vi "Parse JSON Item.vi"(8 "error in (no error)":errorcluster, 9 "Name":string, 10 "Variant in":variant, 11 "JSON In":string) -> (0 "error out":errorcluster, 2 "Variant out":variant)   [LabVIEW 2018]
uses:
  a599c9c2-7984-4765-8e85-315dde484629.vi
  <vilib>/JDP Science/JSONtext/Next JSON Value.vi
  <vilib>/JDP Science/JSONtext/String Subset.vi
  <vilib>/JDP Science/JSONtext/Parsing/Advance past next JSON Value (inlined COPY).vi
  <vilib>/JDP Science/JSONtext/Parsing/Advance past whitespace.vi
  <vilib>/JDP Science/JSONtext/Parsing/Advance past String.vi
  <vilib>/JDP Science/JSONtext/Parsing/Advance past Number.vi
  <vilib>/JDP Science/JSONtext/Parsing/Advance past Line Ending.vi
  <vilib>/JDP Science/JSONtext/Parsing/Parse Full Path or Item Name.vi
  <vilib>/JDP Science/JSONtext/Parsing/Advance past Array.vi
  <vilib>/JDP Science/JSONtext/Parsing/Advance past Object.vi
  <vilib>/JDP Science/JSONtext/support/Error Cluster From Code.vi
  <vilib>/JDP Science/JSONtext/Offset/Find Item Locations by Path.vi
  <vilib>/JDP Science/JSONtext/JSON text to Variant.vi
  <vilib>/JDP Science/JSONtext/LVClass Serializer/JSONtext LVClass Serializer.lvclass
  <vilib>/JDP Science/JSONtext/JSONtext.lvlib
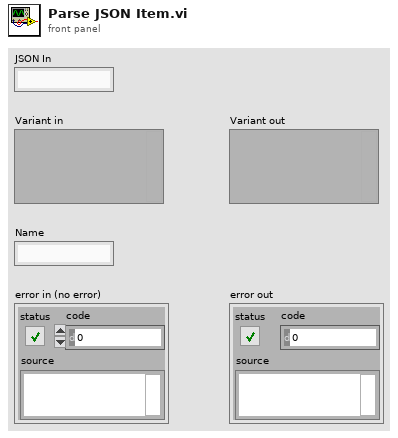
[diagram p1: front panel]
types:
  T1 = typedef "JSONtext.lvlib/JSON Value Type.ctl" = enum16{"Not a JSON Value", "JSON Object", "JSON Array", "String", "Number", "true", "false", "null"}
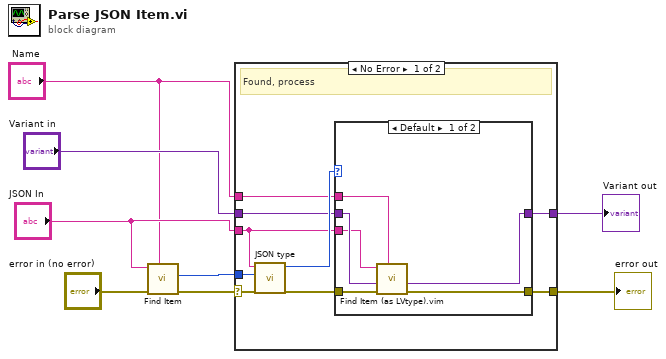
[diagram p0: block diagram]
diagram:
  n1 = call <vilib>:"Find Item.vi"("$Path or Item Name"="Name", "error in (no error)"="error in (no error)", "JSON"="JSON In") -> ("error out"=w5:errorcluster, "Item offset"=w3:i32)  [unwired: 5 in, 2 out]
  n2 = case shown="No Error" w5 {
    selector: w5 -> [w14 w25]
    tunnel: "JSON In" -> [w9 _]
    tunnel: w3 -> [w16 _]
    tunnel: "Variant in" -> [w13 w26]
    tunnel: "Name" -> [w12 _]
    tunnel: [w11 w26] -> w6
    tunnel: [w10 w25] -> w7
    frame No Error {
      # "Found, process"
      n3 = call <vilib>:"JSON type.vi"("Offset"=w16, "JSON"=w9) -> ("JSON Value Type"=w15:T1)  [unwired: 8 in, 1 out]
      n4 = case shown="Default" w15 {
        tunnel: w14 -> [w22 w23]
        tunnel: w13 -> [w21 w24]
        tunnel: w12 -> [w20 _]
        tunnel: [w19 w24] -> w11
        tunnel: [w18 w23] -> w10
        tunnel: w9 -> [w17 _]
        frame Default {
          n5 = call "Find Item (as LVtype).vim"("$Path or Item Name"=w20, "error in (no error)"=w22, "Data Type and Default Value"=w21, "JSON"=w17) -> ("error out"=w18:errorcluster, "Data"=w19:variant)  [unwired: 4 in, 2 out]
        }
        frame "Not a JSON Value", "null" {
        }
      }
    }
    frame Error {
      # "Not Found"
    }
  }
  "error out" <- w7
  "Variant out" <- w6
